vi "Teleop.vi"(10 "Match Info":T1={"Autonomous Elapsed Seconds"=0.0, "TeleOp Elapsed Seconds"=0.0, "Disabled Elapsed Seconds"=0.0, "Visited Autonomous"=FALSE, "Visited TeleOp"=FALSE, "Visited Disabled"=FALSE, "Autonomous Settings"={"Autonomous Style"=enum."Independent", "VI Refnum"=refnum}}, 11 "Call Context":T2) -> ()   [LabVIEW 2017]
doc: "This VI is called for each enabled TeleOp packet received from the DS. It is typically used to read from joysticks and other inputs and update I/O or setpoints for timed control loops. It should complete and return within 20 milliseconds or risk missing DS packets."
uses:
  <vilib>/Rock Robotics/WPI/DriverStation/WPI_DriverStationDerivedRobotMode.ctl
  <vilib>/Rock Robotics/WPI/DriverStation/WPI_DriverStationMatch Info.ctl
  <vilib>/Rock Robotics/WPI/Utilities/WPI_GetSetVariantRefNum.vi
  <vilib>/Rock Robotics/Network Tables/NT Write Numeric Array.vi
  <vilib>/Rock Robotics/Network Tables/NT Write Boolean Array.vi
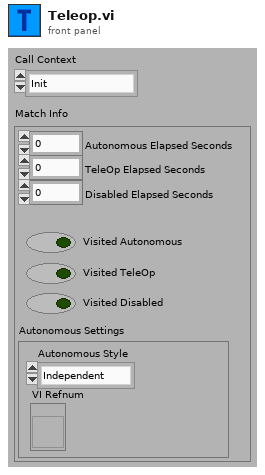
[diagram p1: front panel]
types:
  T1 = typedef "WPI_DriverStationMatch Info.ctl" = cluster{"Autonomous Elapsed Seconds":dbl, "TeleOp Elapsed Seconds":dbl, "Disabled Elapsed Seconds":dbl, "Visited Autonomous":bool, "Visited TeleOp":bool, "Visited Disabled":bool, "Autonomous Settings":cluster{"Autonomous Style":enum16{"Iterative", "Independent"}, "VI Refnum":refnum<vi>}}
  T2 = typedef "WPI_DriverStationDerivedRobotMode.ctl" = enum16{"Init", "Execute", "Stop"}
  T3 = typedef "WPI_JoystickDevRef.ctl" = cluster{"Device":T4}
  T4 = typedef "WPI_JoystickDeviceEnum.ctl" = enum16{"USB 0", "USB 1", "USB 2", "USB 3", "USB 4", "USB 5"}
  T5 = enum16{"Linear", "Square  Root", "Square", "n^x"}
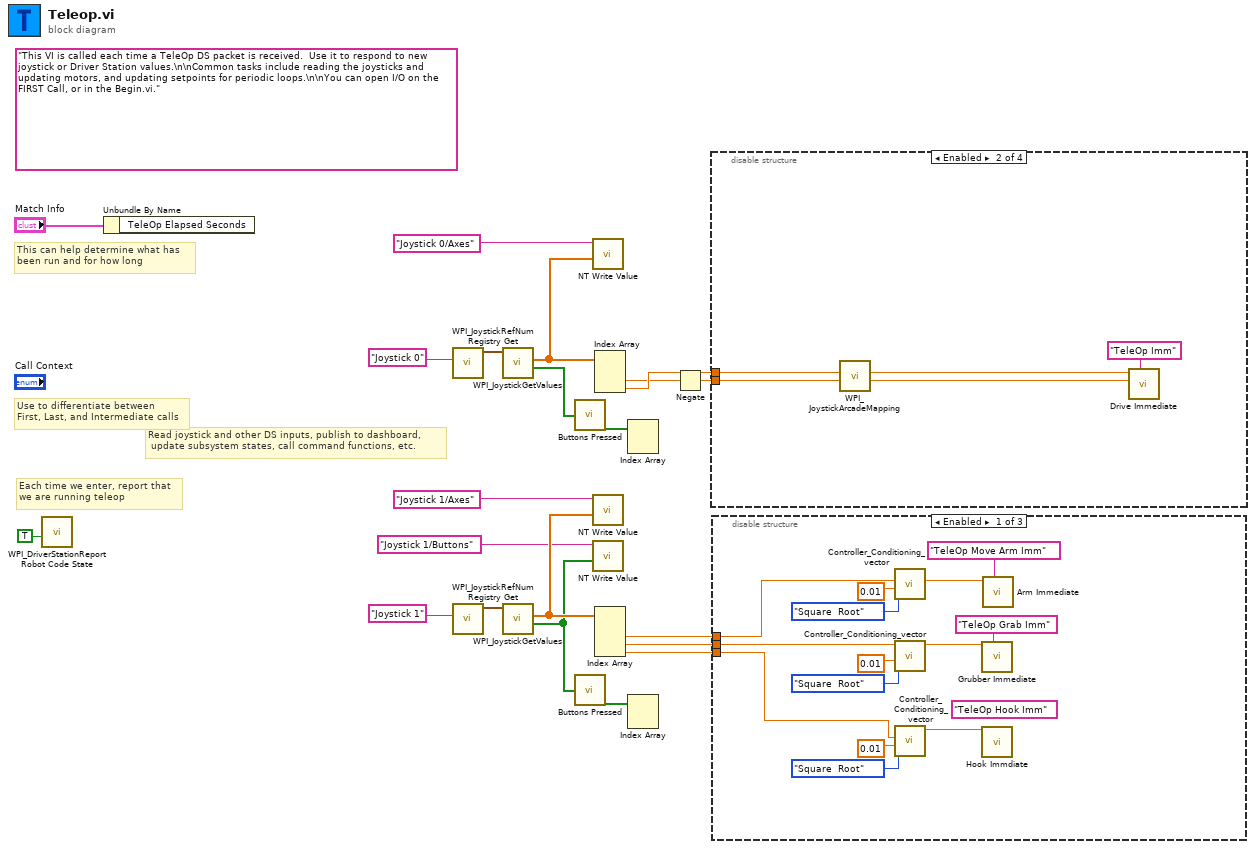
[diagram p0: block diagram]
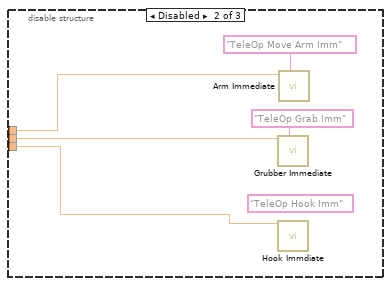
[diagram p2: hidden frame]
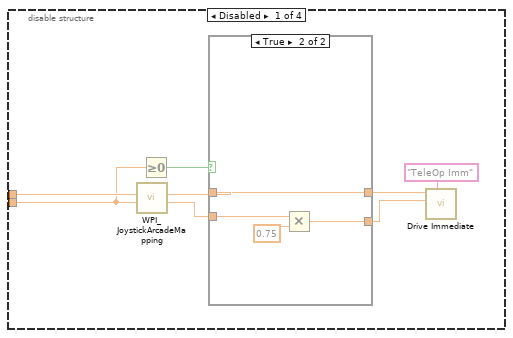
[diagram p4: hidden frame]
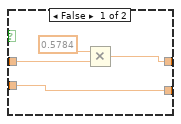
[diagram p5: hidden frame]
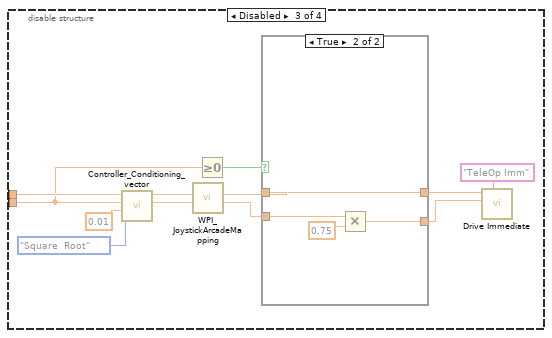
[diagram p6: hidden frame]
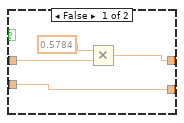
[diagram p7: hidden frame]
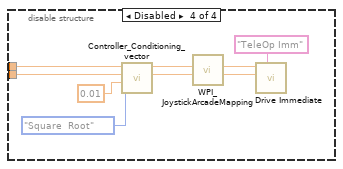
[diagram p8: hidden frame]
diagram:
  (unwired) "This VI is called each time a TeleOp DS packet is received.  Use it to respond to new joystick or Driver Station values.\n\nCommon tasks include reading the joysticks and updating motors, and updating setpoints for periodic loops.\n\nYou can open I/O on the FIRST Call, or in the Begin.vi."
  # "Read joystick and other DS inputs, publish to dashboard,\n update subsystem states, call command functions, etc."
  # "Each time we enter, report that\nwe are running teleop"
  # "Use to differentiate between\nFirst, Last, and Intermediate calls"
  # "This can help determine what has\nbeen run and for how long"
  n1 = call <vilib>:"WPI_DriverStationReport Robot Code State.vi"("TeleOp"=TRUE ("Autonomous")) -> ()  [unwired: 10 in, 1 out]
  n2 = Unbundle By Name("Match Info") -> ()  [unwired: 1 out]
  n3 = call <vilib>:"WPI_JoystickRefNum Registry Get.vi"("refnum name"="Joystick 0") -> ("JoystickDevRef"=w18:T3)  [unwired: 1 in, 9 out]
  n4 = call <vilib>:"WPI_JoystickRefNum Registry Get.vi"("refnum name"="Joystick 1") -> ("JoystickDevRef"=w5:T3)  [unwired: 1 in, 9 out]
  n5 = call <vilib>:"WPI_JoystickGetValues.vi"("JoystickDevRef"=w18) -> ("Buttons"=w16:bool[], "Axes"=w15:dbl[])  [unwired: 6 in, 3 out]
  n6 = call <vilib>:"WPI_JoystickGetValues.vi"("JoystickDevRef"=w5) -> ("Buttons"=w8:bool[], "Axes"=w9:dbl[])  [unwired: 6 in, 3 out]
  n7 = call "Buttons Pressed.vi"("Button Values"=w16) -> ("Button Presses"=w17:bool[])
  n8 = call "Buttons Pressed.vi"("Button Values"=w8) -> ("Button Presses"=w6:bool[])
  n9 = call-poly <vilib>:"NT Write Value.vi"("Numeric Array"=w15, "Name"="Joystick 0/Axes") -> ()  [unwired: 9 in, 1 out]
  n10 = call-poly <vilib>:"NT Write Value.vi"("Numeric Array"=w9, "Name"="Joystick 1/Axes") -> ()  [unwired: 9 in, 1 out]
  n11 = call-poly <vilib>:"NT Write Value.vi"("Boolean Array"=w8, "Name"="Joystick 1/Buttons") -> ()  [unwired: 9 in, 1 out]
  n12 = Index Array(array=w15) -> (element #2=w12:dbl, element #3=w13:dbl)  [unwired: 3 in, 1 out]
  n13 = Index Array(array=w9) -> (element #2=w3:dbl, element #3=w2:dbl, element #4=w1:dbl)  [unwired: 4 in, 1 out]
  n14 = Index Array(array=w17) -> ()  [unwired: 2 in, 2 out]
  n15 = Index Array(array=w6) -> ()  [unwired: 2 in, 2 out]
  n16 = Negate(x=w12) -> (-x=w11:dbl)
  n17 = disable-structure shown="Enabled" {
    disable-tunnel: w13 -> [w28 w41 w46 w66]
    disable-tunnel: w11 -> [w22 w38 w45 w65]
    frame Disabled {
      n18 = call <vilib>:"WPI_JoystickArcadeMapping.vi"("Y axis value"=w22, "X axis value"=w28) -> ("Right Motor Value"=w25:dbl, "Left Motor Value"=w26:dbl)  [unwired: 8 in]
      n19 = Greater Or Equal To 0?(x=w22) -> (x >= 0?=w27:bool)
      n20 = case shown="True" w27 {
        tunnel: w26 -> [w33 w37]
        tunnel: [w32 w37] -> w24
        tunnel: w25 -> [w30 w36]
        tunnel: [w30 w34] -> w23
        frame False {
          n21 = Multiply(x=0.5784, y=w33) -> (x*y=w32:dbl)
        }
        frame True {
          n22 = Multiply(x=w36, y=0.75) -> (x*y=w34:dbl)
        }
      }
      n23 = call "Drive Immediate.vi"("Description"="TeleOp Imm", "Right Setpoint"=w23, "Left Setpoint"=w24) -> ()  [unwired: 8 in, 1 out]
    }
    frame Enabled {
      n24 = call <vilib>:"WPI_JoystickArcadeMapping.vi"("Y axis value"=w38, "X axis value"=w41) -> ("Right Motor Value"=w39:dbl, "Left Motor Value"=w40:dbl)  [unwired: 8 in]
      n25 = call "Drive Immediate.vi"("Description"="TeleOp Imm", "Right Setpoint"=w39, "Left Setpoint"=w40) -> ()  [unwired: 8 in, 1 out]
    }
    frame Disabled {
      n26 = call "Controller_Conditioning_vector.vi"("Enum"=T5."Square  Root", "Dead Zone(0 to 1)"=0.01, "Y(-1 to 1)"=w45, "X(-1 to 1)"=w46) -> ("Y"=w43:dbl, "X"=w44:dbl)  [unwired: 4 in, 2 out]
      n27 = call <vilib>:"WPI_JoystickArcadeMapping.vi"("Y axis value"=w43, "X axis value"=w44) -> ("Right Motor Value"=w51:dbl, "Left Motor Value"=w52:dbl)  [unwired: 8 in]
      n28 = Greater Or Equal To 0?(x=w45) -> (x >= 0?=w53:bool)
      n29 = case shown="True" w53 {
        tunnel: w52 -> [w58 w62]
        tunnel: [w57 w62] -> w50
        tunnel: w51 -> [w55 w61]
        tunnel: [w55 w59] -> w49
        frame False {
          n30 = Multiply(x=0.5784, y=w58) -> (x*y=w57:dbl)
        }
        frame True {
          n31 = Multiply(x=w61, y=0.75) -> (x*y=w59:dbl)
        }
      }
      n32 = call "Drive Immediate.vi"("Description"="TeleOp Imm", "Right Setpoint"=w49, "Left Setpoint"=w50) -> ()  [unwired: 8 in, 1 out]
    }
    frame Disabled {
      n33 = call "Controller_Conditioning_vector.vi"("Enum"=T5."Square  Root", "Dead Zone(0 to 1)"=0.01, "Y(-1 to 1)"=w65, "X(-1 to 1)"=w66) -> ("Y"=w63:dbl, "X"=w64:dbl)  [unwired: 4 in, 2 out]
      n34 = call <vilib>:"WPI_JoystickArcadeMapping.vi"("Y axis value"=w63, "X axis value"=w64) -> ("Right Motor Value"=w69:dbl, "Left Motor Value"=w70:dbl)  [unwired: 8 in]
      n35 = call "Drive Immediate.vi"("Description"="TeleOp Imm", "Right Setpoint"=w69, "Left Setpoint"=w70) -> ()  [unwired: 8 in, 1 out]
    }
  }
  n36 = disable-structure shown="Enabled" {
    disable-tunnel: w3 -> [w80 w88 _]
    disable-tunnel: w2 -> [w79 w87 _]
    disable-tunnel: w1 -> [w72 w86 _]
    frame Enabled {
      (unwired) "TeleOp Hook Imm" ("Description")
      n37 = call "Controller_Conditioning_vector.vi"("Enum"=T5."Square  Root", "Dead Zone(0 to 1)"=0.01, "Y(-1 to 1)"=w80) -> ("Y"=w83:dbl)  [unwired: 5 in, 3 out]
      n38 = call "Controller_Conditioning_vector.vi"("Enum"=T5."Square  Root", "Dead Zone(0 to 1)"=0.01, "X(-1 to 1)"=w79) -> ("X"=w78:dbl)  [unwired: 5 in, 3 out]
      n39 = call "Controller_Conditioning_vector.vi"("Enum"=T5."Square  Root", "Dead Zone(0 to 1)"=0.01, "Y(-1 to 1)"=w72) -> ("X"=w75:dbl)  [unwired: 5 in, 3 out]
      n40 = call "Grubber Immediate.vi"("Description"="TeleOp Grab Imm", "Setpoint"=w78) -> ()  [unwired: 9 in, 1 out]
      n41 = call "Hook Immdiate.vi"("Setpoint"=w75) -> ()  [unwired: 10 in, 1 out]
      n42 = call "Arm Immediate.vi"("Description"="TeleOp Move Arm Imm", "Setpoint"=w83) -> ()  [unwired: 9 in, 1 out]
    }
    frame Disabled {
      (unwired) "TeleOp Hook Imm" ("Description")
      n43 = call "Grubber Immediate.vi"("Description"="TeleOp Grab Imm", "Setpoint"=w87) -> ()  [unwired: 9 in, 1 out]
      n44 = call "Hook Immdiate.vi"("Setpoint"=w86) -> ()  [unwired: 10 in, 1 out]
      n45 = call "Arm Immediate.vi"("Description"="TeleOp Move Arm Imm", "Setpoint"=w88) -> ()  [unwired: 9 in, 1 out]
    }
    frame Disabled {
    }
  }
